vi "Modify Software Feed.vi"(5 "New Feed Name":string, 6 "Trusted (F)":bool, 7 "Enabled (T)":bool=TRUE, 8 "error in (no error)":errorcluster, 9 "URI":string, 10 "Feed Name":string, 11 "Session in":refnum<k21>) -> (0 "error out":errorcluster, 3 "Session out":refnum<k21>)   [LabVIEW 2017, in "nisyscfg.lvlib"]
doc: "Modifies an existing software feed by name. This requires Secure Shell Server (sshd) to be enabled on the target."
uses:
  <vilib>/nisyscfg/nisyscfg.lvlib
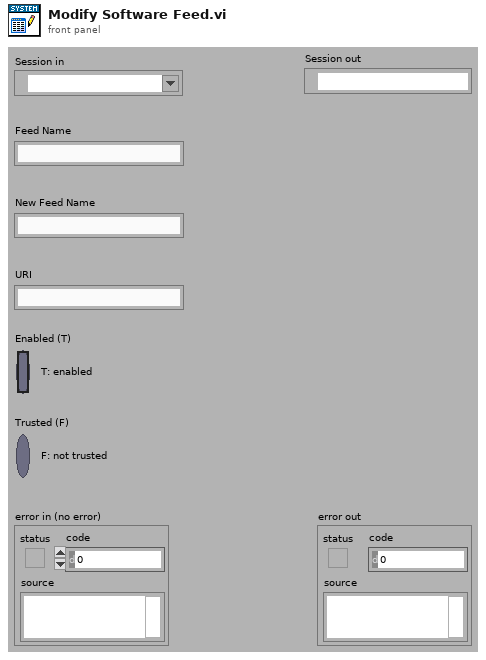
[diagram p1: front panel]
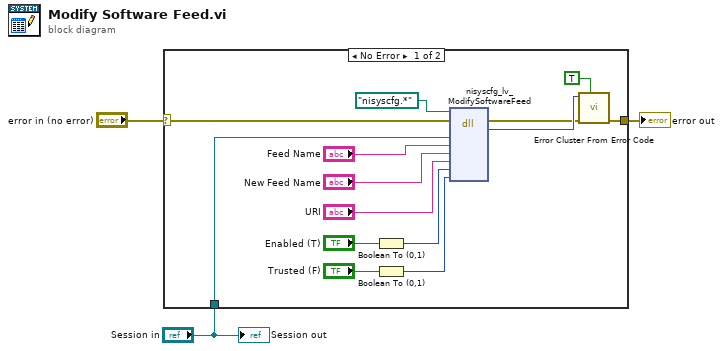
[diagram p0: block diagram]
diagram:
  n1 = case shown="No Error" "error in (no error)" {
    selector: "error in (no error)" -> [w12 w18]
    tunnel: [w13 w18] -> w3
    tunnel: "Session in" -> [w5 _]
    frame No Error {
      n2 = Boolean To (0,1)(Boolean="Enabled (T)") -> (0, 1=w9:i16)
      n3 = Boolean To (0,1)(Boolean="Trusted (F)") -> (0, 1=w8:i16)
      n4 = dll-call lib="nisyscfg.*" fn="nisyscfg_lv_ModifySoftwareFeed" label="ModifySoftwareFeed"(path in=path "nisyscfg.*", error in=w12, "sessionHandle"=w5, "feedName"="Feed Name", "newFeedName"="New Feed Name", "uri"="URI", "enabled"=w9, "trusted"=w8) -> (error out=w16:errorcluster, "return type"=w17:i32)  [unwired: 7 in, 1 out]
      n5 = call <vilib>:"Error Cluster From Error Code.vi"("show call chain? (False)"=TRUE, "error in (no error)"=w16, "error code (0)"=w17) -> ("error out"=w13:errorcluster)  [unwired: 6 out]
    }
    frame Error {
    }
  }
  "error out" <- w3
  "Session out" <- "Session in"
